vi "sub_SDR_demod_QAM64.vi"(11 "Input Symbols":cdb[](array[numeric])) -> (3 "Demodulated data":bool[](array[boolean]))   [LabVIEW 2012]
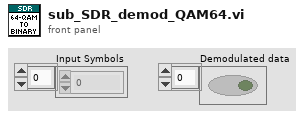
[diagram p1: front panel]
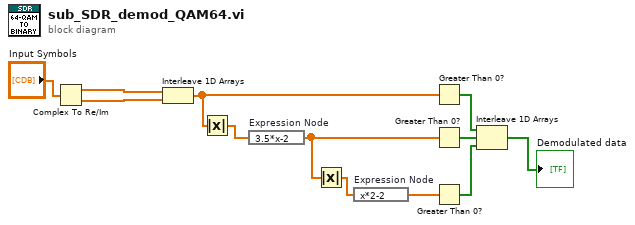
[diagram p0: block diagram]
diagram:
  n1 = Complex To Re/Im(x + iy="Input Symbols") -> (x=w1:dbl[], y=w2:dbl[])
  n2 = Interleave 1D Arrays "Interleave 1D Arrays"(w1, w2) -> (w10:dbl[])
  n3 = Absolute Value(x=w10) -> (abs(x)=w5:dbl[])
  n4 = expression code="3.5*x-2"(w5) -> (w4:dbl[])
  n5 = Absolute Value(x=w4) -> (abs(x)=w6:dbl[])
  n6 = expression code="x*2-2"(w6) -> (w3:dbl[])
  n7 = Greater Than 0?(x=w10) -> (x > 0?=w9:bool[])
  n8 = Greater Than 0?(x=w4) -> (x > 0?=w8:bool[])
  n9 = Greater Than 0?(x=w3) -> (x > 0?=w7:bool[])
  n10 = Interleave 1D Arrays "Interleave 1D Arrays"(w9, w8, w7) -> (→"Demodulated data":bool[])
